vi "STM Set Meta Data (UDP Clst).vi"(7 "Meta data":T2[](array[typedef]), 8 "error in":errorcluster, 11 "Connection Info":T1) -> (0 "error out":errorcluster, 3 "Connection Info Out":T1)   [LabVIEW 2014, in "QwaveSys Raspberry Pi Library.lvlib"]
doc: "Assigns the meta data cluster associated with this STM session."
uses:
  QwaveSys Raspberry Pi Library.lvlib
  stm_UDP Connection Info.ctl
  _SubVIs/stm_MetaDataElement.ctl
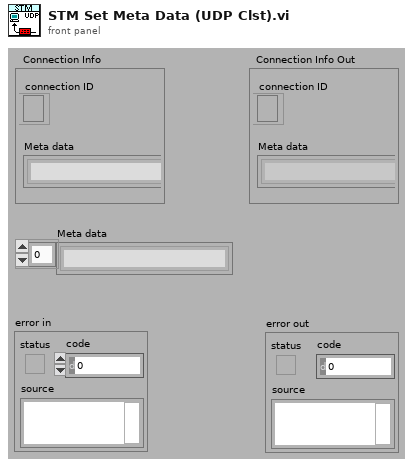
[diagram p1: front panel]
types:
  T1 = typedef "QwaveSys Raspberry Pi Library.lvlib/stm_UDP Connection Info.ctl" = cluster{"connection ID":refnum<k16>, "Meta data":T2[]}
  T2 = typedef "QwaveSys Raspberry Pi Library.lvlib/stm_MetaDataElement.ctl" = string
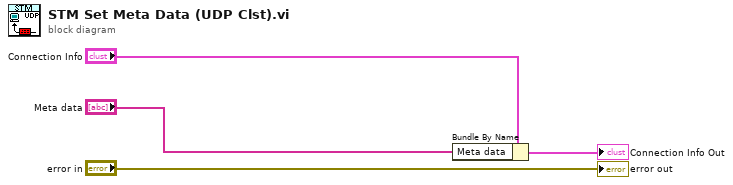
[diagram p0: block diagram]
diagram:
  n1 = Bundle By Name(cluster="Connection Info", "Meta data"="Meta data") -> (→"Connection Info Out":T1)
  "error out" <- "error in"
